vi "Set App View.vi"(8 "error in (no error)":errorcluster, 11 "menu reference":refnum<k9>) -> (0 "error out":errorcluster)   [LabVIEW 2024, in "User Interface.lvlib"]
uses:
  User Interface.lvlib
  Support/General Type Defs/Global Data.vi
  UI Queue - Enqueue.vi
  Support/General Type Defs/General Type Definitions.lvlib
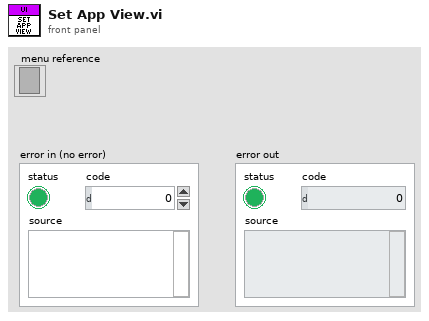
[diagram p1: front panel]
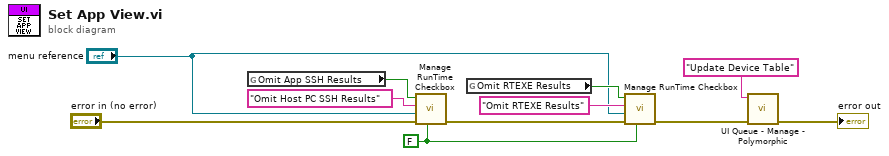
[diagram p0: block diagram]
diagram:
  w7 = FALSE ("Set(T)/Get(F)")
  n1 = global read "Global Data.vi" "Omit App SSH Results"() -> (w2:bool)
  n2 = call "Manage RunTime Checkbox.vi"("Change(T)/set(F)"=w7, "error in (no error)"="error in (no error)", "Message Data"="menu reference", "String"="Omit Host PC SSH Results" ("Message"), "Menu Checkbox"=w2) -> ("error out"=w8:errorcluster)  [unwired: 5 in, 1 out]
  n3 = global read "Global Data.vi" "Omit RTEXE Results"() -> (w5:bool)
  n4 = call "Manage RunTime Checkbox.vi"("Change(T)/set(F)"=w7, "error in (no error)"=w8, "Message Data"="menu reference", "String"="Omit RTEXE Results" ("Message"), "Menu Checkbox"=w5) -> ("error out"=w1:errorcluster)  [unwired: 5 in, 1 out]
  n5 = call-poly "UI Queue - Manage - Polymorphic.vi"("error in"=w1, "Message"="Update Device Table") -> ("error out"=→"error out":errorcluster)  [unwired: 9 in]
